vi "Main.vi"() -> ()   [LabVIEW 2017]
doc: "The program is for the real-time control of digital output pins on the Arduino Uno microcontroller.\n\nThe program is configured for the use of 6 DIO pins numbered 2-7. The pins can be be used to output AC and DC signals. The pins can also be swtiched on for a preset length of time."
uses:
  controls/UI Data.ctl
  <vilib>/MakerHub/LINX/Public/Peripherals/Digital/Digital Write 1 Chan.vi
  <vilib>/MakerHub/LINX/Public/Peripherals/Digital/Digital Write N Chans.vi
  <vilib>/MakerHub/LINX/Private/Local IO/LinxDigitalWrite.vi
  <vilib>/MakerHub/LINX/Public/Utilities/Check Channel.vi
  support/Message Queue/Enqueue Message (Single).vi
  <vilib>/MakerHub/LINX/Public/Utilities/Open Serial.vi
  <vilib>/MakerHub/LINX/Private/Utilties/Generate Error.vi
  <vilib>/Utility/error.llb/Error Cluster From Error Code.vi
  <vilib>/ErrorRing/Error Ring.xnode
  support/Message Queue/Message Queue.lvlib
  support/User Event - Stop/User Event - Stop.lvlib
  <vilib>/MakerHub/LINX/LMH-LINX.lvlib
panel:
  in  "Data Buffer":u64
  out "Playing Record":bool
  in  "Record New Sequence":bool
  in  "Play Button":bool
  in  "Previous Button":bool
  in  "Stop Button":bool
  in  "Next Button":bool
  in  "LG Electrodes":bool[][](array[boolean])=[[FALSE, FALSE], [FALSE, FALSE], [FALSE, FALSE]]
  in  "SM Electrodes":bool[][](array[boolean])=[[FALSE, FALSE, FALSE, FALSE, FALSE, FALSE], [FALSE, FALSE, FALSE, FALSE, FALSE, FALSE], [FALSE, FALSE, FALSE, FALSE, FALSE, FALSE], [FALSE, FALSE, FALSE, FALSE, FALSE, FALSE], [FALSE, FALSE, FALSE, FALSE, FALSE, FALSE], [FALSE, FALSE, FALSE, FALSE, FALSE, FALSE]]
  in  "XS Electrodes":bool[][](array[boolean])=[[FALSE, FALSE, FALSE], [FALSE, FALSE, FALSE], [FALSE, FALSE, FALSE], [FALSE, FALSE, FALSE], [FALSE, FALSE, FALSE], [FALSE, FALSE, FALSE]]
  in  "Frequency (Hz)":dbl
  in  "DC/AC":bool
  in  "On-time (ms)":dbl
  in  "Start Button":bool
  in  "COM Port":refnum<visa-resource-name>="COM3"
  out "User Prompts":string="Initializing...."
  in  "Restart Button":bool
  in  "Exit":bool
  # "Digital Microfluidics HV Switching Control"
  # "Electrode Recorded Sequence"
  # "Electrode Controls"
  # "Timing Controls"
  # "DC"
  # "AC"
  # "Program Status"
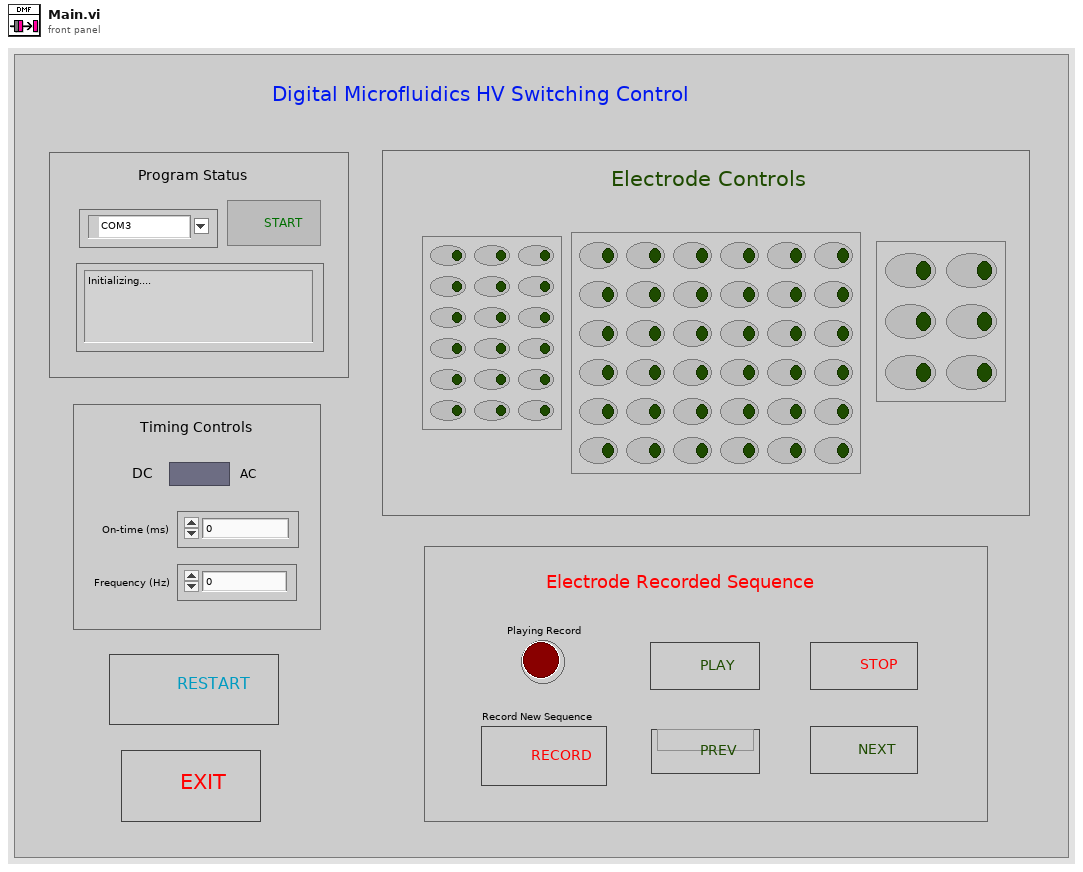
[diagram p1: front panel]
types:
  T1 = typedef "UI Data.ctl" = cluster{"VISA resource name":refnum<vi>, "Start Button":refnum<vi>, "DC/AC":refnum<vi>, "On-time (ms)":refnum<vi>, "Frequency (Hz)":refnum<vi>, "User Prompts":refnum<vi>, "XS Electrodes":refnum<vi>, "SM Electrodes":refnum<vi>, "LG Electrodes":refnum<vi>, "Data Buffer":refnum<vi>, "Play Button":refnum<vi>, "Playing Record":refnum<vi>, "Restart Button":refnum<vi>, "Exit":refnum<vi>}
  T2 = typedef "Message Queue.lvlib/All Message Queues.ctl" = cluster{"UI":refnum<queue>}
  T3 = typedef "LMH-LINX.lvlib/LINX Ref.ctl" = cluster{"IO":T4, "Interface":T5, "LINX Device Config":T6}
  T4 = typedef "LMH-LINX.lvlib/Platform.ctl" = enum16{"Remote", "Local"}
  T5 = typedef "LMH-LINX.lvlib/Interface.ctl" = enum16{"Serial", "TCP"}
  T6 = typedef "LMH-LINX.lvlib/Device.lvlib/LINX Device Config.ctl" = cluster{"Interface":T5, "COM Port":refnum<visa-resource-name>, "TCP Configuration":T7, "Device Family":u8, "Device ID":u8, "Device Name":string, "TCP Ref":refnum<k5>, "Channels":T8}
  T7 = typedef "LMH-LINX.lvlib/Device.lvlib/TCP Config.ctl" = cluster{"IP Address":string, "Port":u16}
  T8 = typedef "LMH-LINX.lvlib/Channels.ctl" = cluster{"DI":u8[], "DO":u8[], "AI":u8[], "AO":u8[], "PWM":u8[], "QE":u8[], "UART":u8[], "I2C 2":u8[], "SPI":u8[], "CAN":u8[], "Servo":u8[], "AI Ref (V)":dbl, "AI Resolution (Bits)":u8, "AO Ref (V)":dbl, "AO Resolution (Bits)":u8}
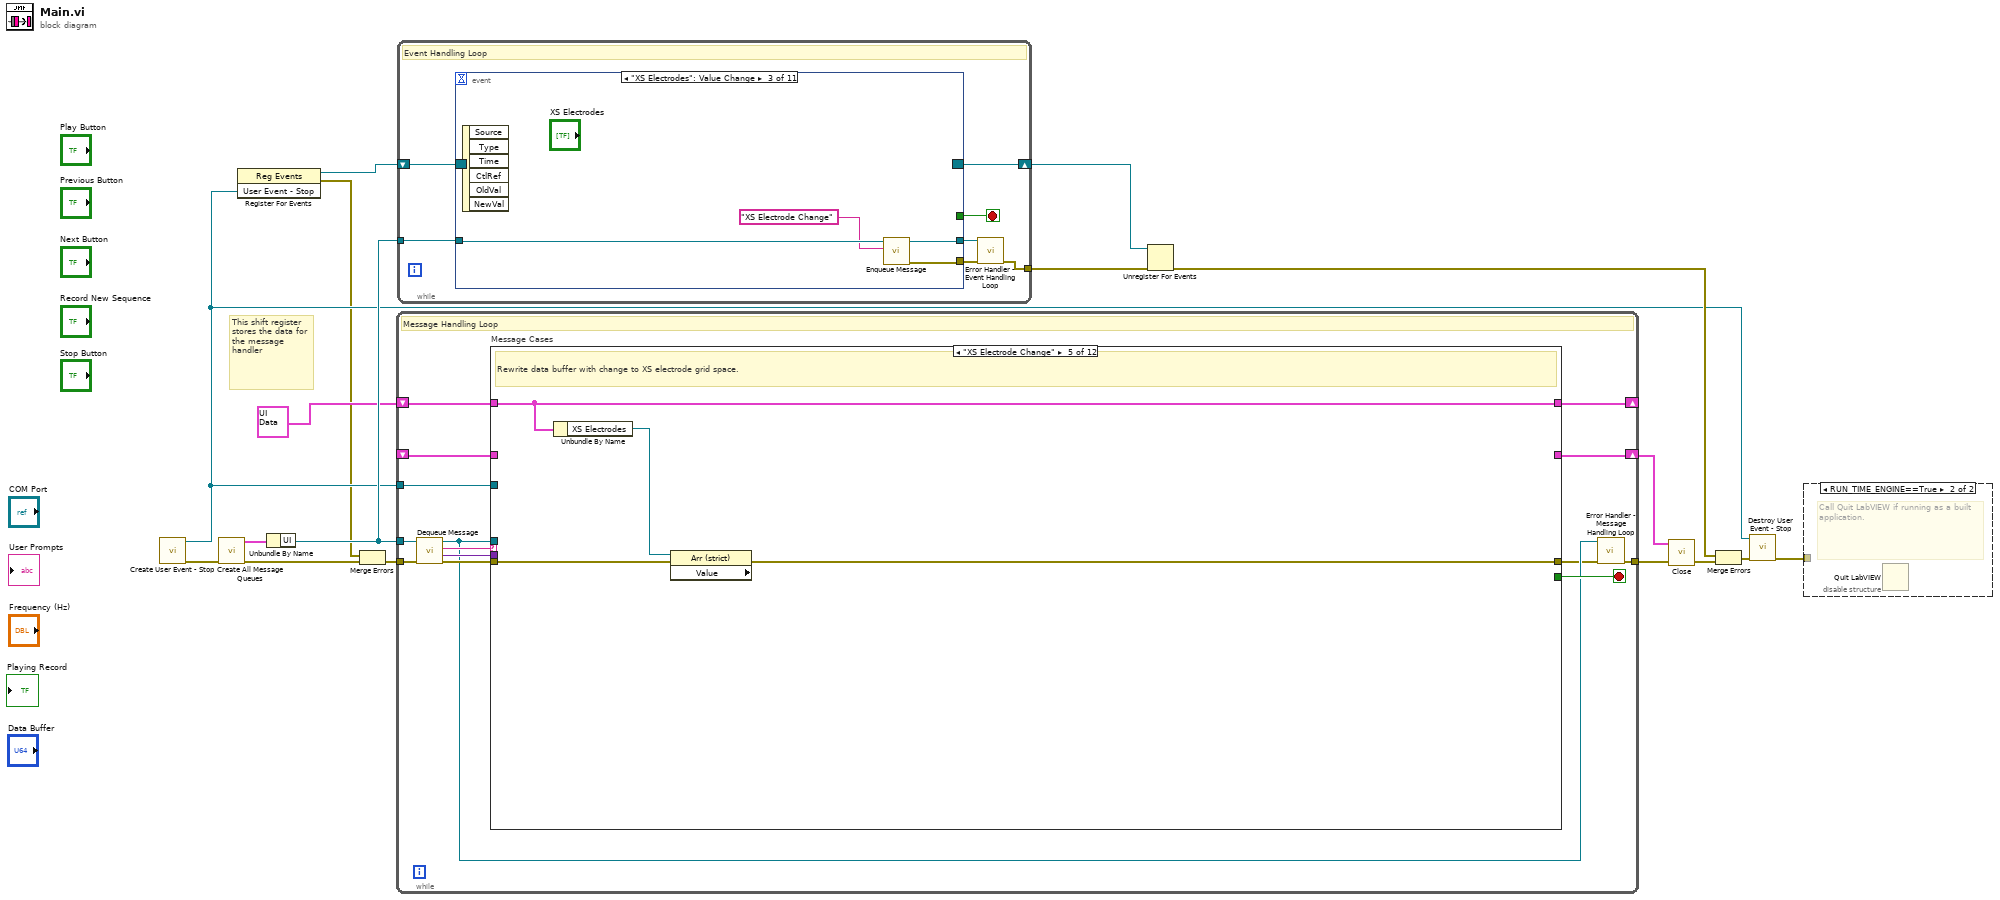
[diagram p0: block diagram]
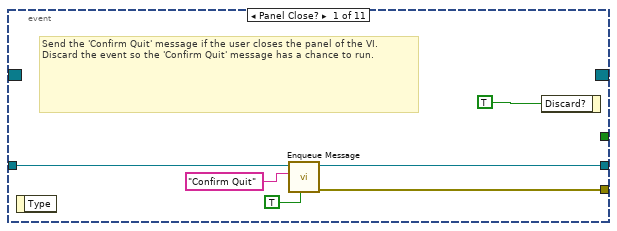
[diagram p3: hidden frame]
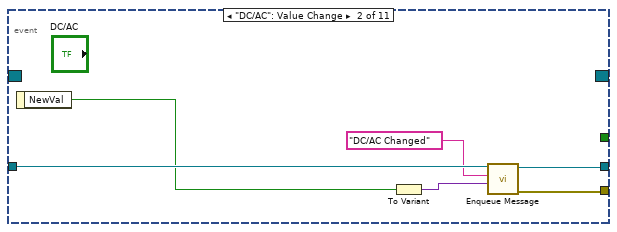
[diagram p4: hidden frame]
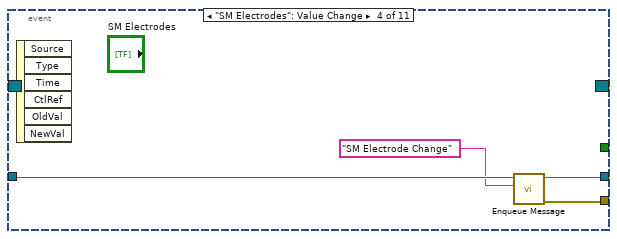
[diagram p5: hidden frame]
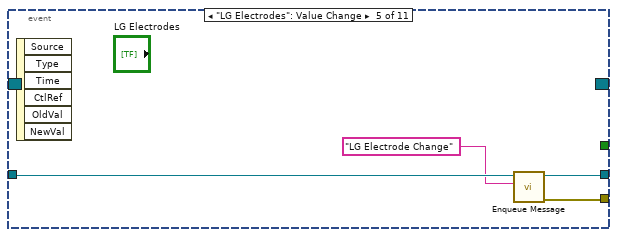
[diagram p6: hidden frame]
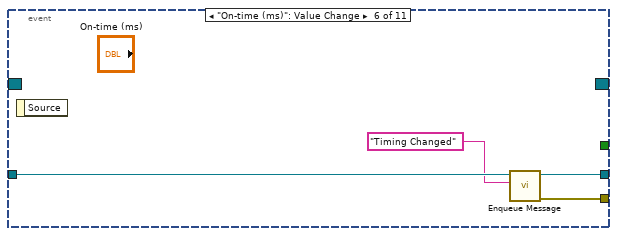
[diagram p7: hidden frame]
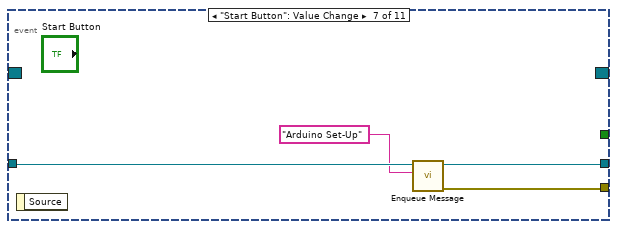
[diagram p8: hidden frame]
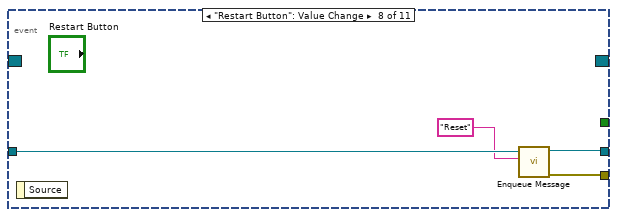
[diagram p9: hidden frame]
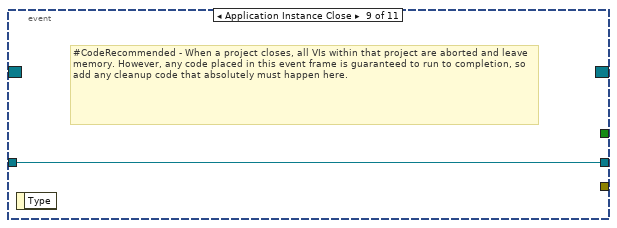
[diagram p10: hidden frame]
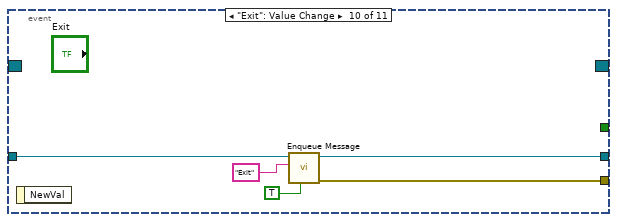
[diagram p11: hidden frame]
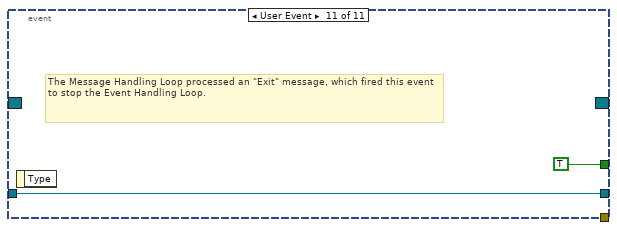
[diagram p12: hidden frame]
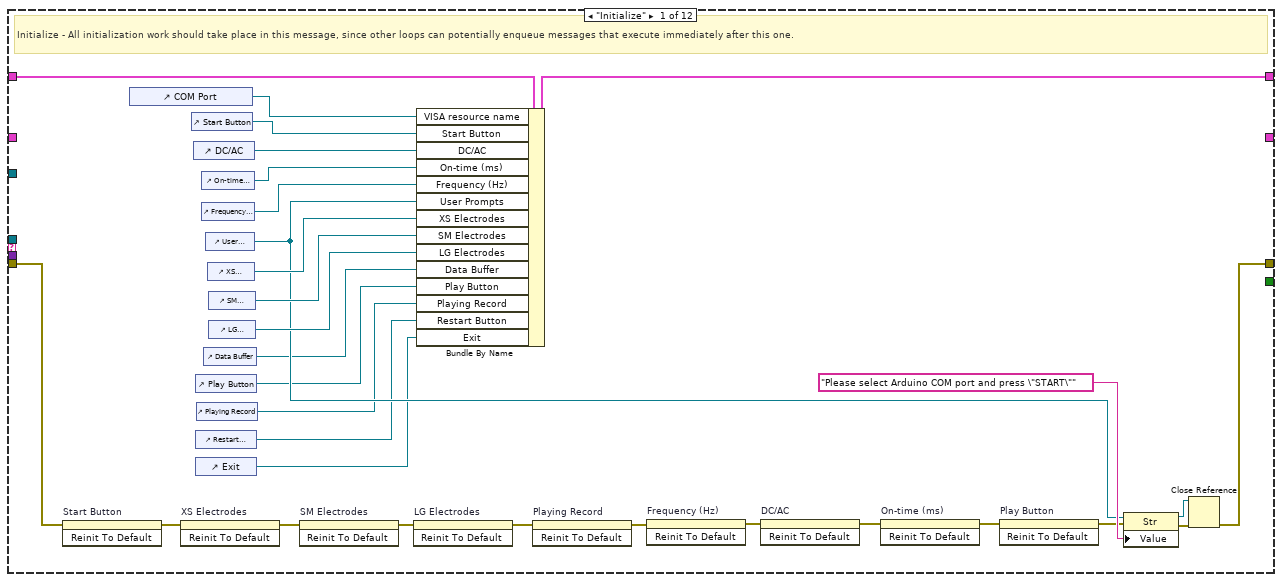
[diagram p13: hidden frame]
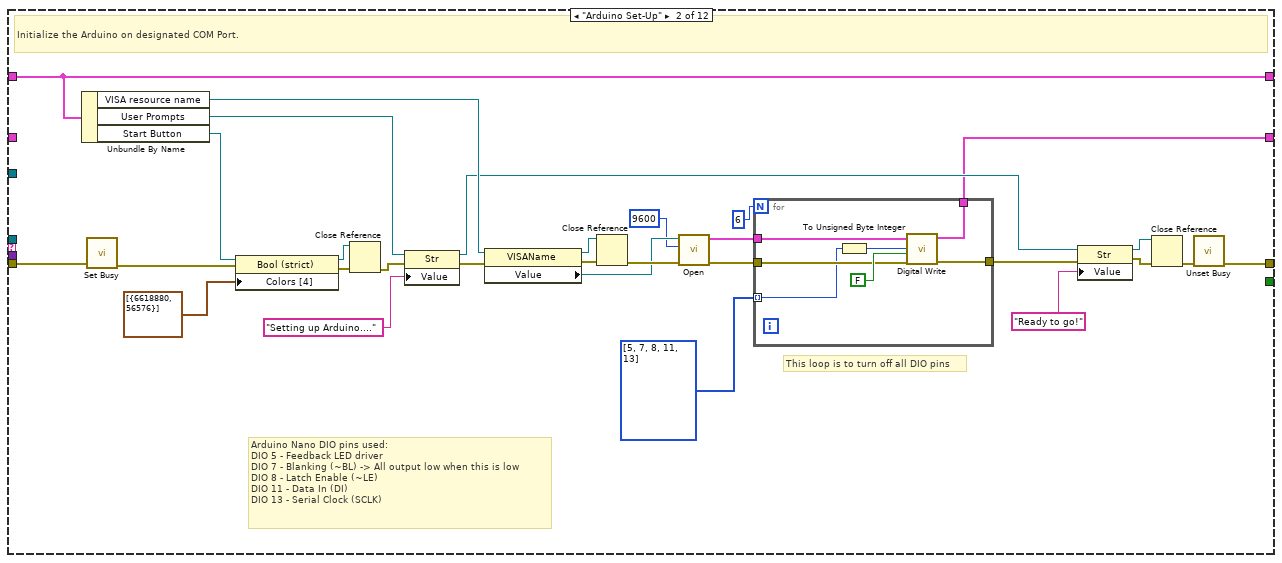
[diagram p14: hidden frame]
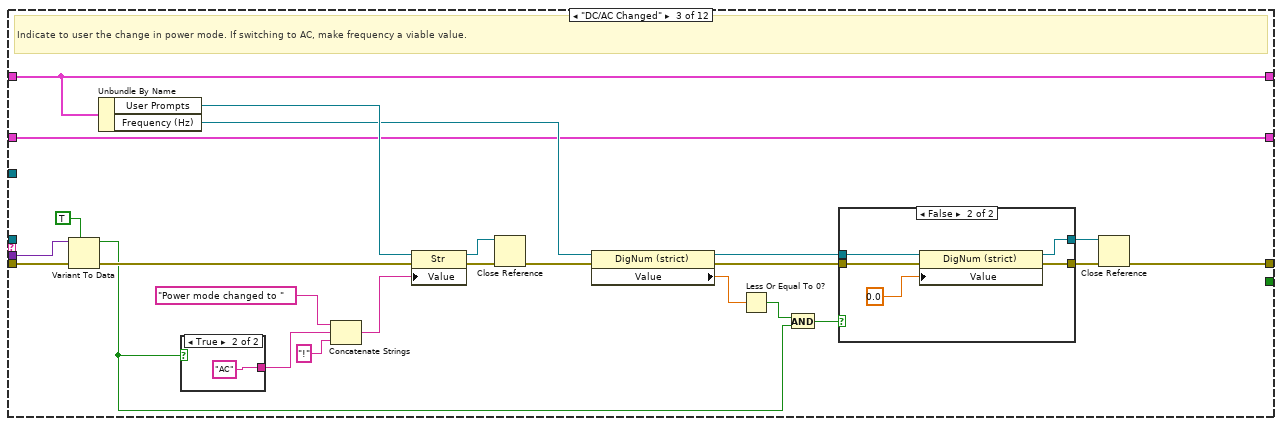
[diagram p15: hidden frame]
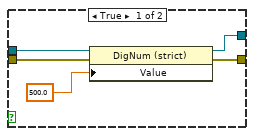
[diagram p16: hidden frame]
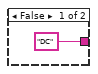
[diagram p17: hidden frame]
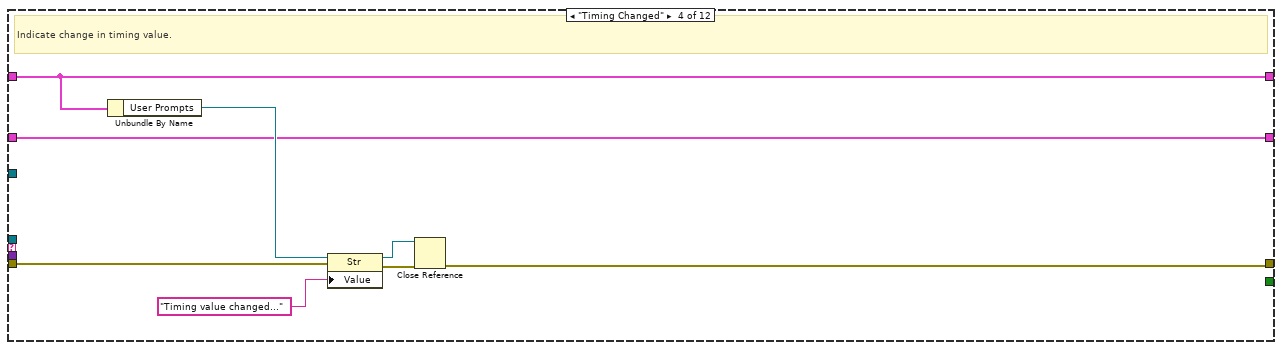
[diagram p18: hidden frame]
diagram:
  # "This shift register stores the data for the message handler"
  n1 = call "Create User Event - Stop.vi"() -> ("error out"=w14:errorcluster, "User Event - Stop"=w7:refnum<user-event>)  [unwired: 10 in]
  n2 = call "Create All Message Queues.vi"("error in (no error)"=w14) -> ("error out"=w17:errorcluster, "Message Queues out"=w16:T2)  [unwired: 9 in]
  n3 = register-events(w7) -> (reference out=w8:refnum<event-registration>, error out=w5:errorcluster)  [unwired: 2 in]
  n4 = Unbundle By Name(w16) -> ("UI"=w15:refnum<queue>)
  n5 = Merge Errors(w5, w17) -> (w6:errorcluster)
  n6 = while {
    tunnel: w15 -> [w23]
    shift-right: [w30] -> _
    shift-left: T1 {"VISA resource name"=refnum, "Start Button"=refnum, "DC/AC"=refnum, "On-time (ms)"=refnum, "Frequency (Hz)"=refnum, "User Prompts"=refnum, "XS Electrodes"=refnum, "SM Electrodes"=refnum, "LG Electrodes"=refnum, "Data Buffer"=refnum, "Play Button"=refnum, "Playing Record"=refnum, "Restart Button"=refnum, "Exit"=refnum} ("Data Cluster") -> [w31]
    tunnel: w7 -> [w28]
    tunnel: w6 -> [w27]
    tunnel: [w21] -> w3
    shift-right: [w19] -> w1
    shift-left: _ -> [w18]
    stop <- w29 stop-if-true
    # "Message Handling Loop"
    n7 = call "Dequeue Message.vi"("error in (no error)"=w27, "Message Queue"=w23) -> ("error out"=w26:errorcluster, "Message Data"=w24:variant, "Message"=w25:string, "dup Message Queue"=w22:refnum<queue>)  [unwired: 6 in]
    n8 = case "Message Cases" shown="\"XS Electrode Change\"" w25 {
      selector: w25 -> [_ _ _ _ _ _ _ _ _ _ _ w218]
      tunnel: w22 -> [_ _ _ _ _ _ _ w161 _ w191 w216 _]
      tunnel: w26 -> [w39 w81 w120 w140 w144 w147 w149 w154 w187 w195 w211 _]
      tunnel: [w55 w79 w100 w136 w142 w147 w149 w162 w181 w193 w214 w219] -> w20
      tunnel: w31 -> [w61 w90 w121 w141 w145 w146 w148 w170 w186 w194 w207 w220]
      tunnel: [w60 w90 w121 w141 w145 w146 w148 w170 w186 w194 w207 w220] -> w30
      tunnel: [_ _ _ _ _ _ _ _ _ _ TRUE _] -> w29
      tunnel: w24 -> [_ _ w119 _ _ _ _ _ w185 _ w208 _]
      tunnel: w28 -> [_ _ _ _ _ _ _ _ _ _ w213 _]
      tunnel: [_ w63 w98 w134 _ _ _ w150 w180 w188 w197 w217] -> w19
      tunnel: w18 -> [_ _ w98 w134 _ _ _ w168 w180 w188 w197 w217]
      frame "Initialize" {
        # "Initialize - All initialization work should take place in this message, since other loops can potentially enqueue messages that execute immediately after this one."
        n9 = invoke on="Start Button" class="Bool (strict)" method="Reinit To Default"(error in=w39) -> (error out=w47:errorcluster)  [unwired: 2 in, 2 out]
        n10 = control-ref of="COM Port"() -> (w59:refnum<vi>)
        n11 = invoke on="XS Electrodes" class="Arr (strict)" method="Reinit To Default"(error in=w47) -> (error out=w46:errorcluster)  [unwired: 2 in, 2 out]
        n12 = control-ref of="Start Button"() -> (w54:refnum<vi>)
        n13 = control-ref of="DC/AC"() -> (w52:refnum<vi>)
        n14 = control-ref of="Play Button"() -> (w35:refnum<vi>)
        n15 = control-ref of="Restart Button"() -> (w33:refnum<vi>)
        n16 = control-ref of="Exit"() -> (w32:refnum<vi>)
        n17 = control-ref of="Playing Record"() -> (w34:refnum<vi>)
        n18 = control-ref of="On-time (ms)"() -> (w51:refnum<vi>)
        n19 = control-ref of="Frequency (Hz)"() -> (w53:refnum<vi>)
        n20 = control-ref of="Data Buffer"() -> (w36:refnum<vi>)
        n21 = control-ref of="User Prompts"() -> (w37:refnum<vi>)
        n22 = control-ref of="XS Electrodes"() -> (w50:refnum<vi>)
        n23 = control-ref of="SM Electrodes"() -> (w49:refnum<vi>)
        n24 = control-ref of="LG Electrodes"() -> (w48:refnum<vi>)
        n25 = invoke on="SM Electrodes" class="Arr (strict)" method="Reinit To Default"(error in=w46) -> (error out=w45:errorcluster)  [unwired: 2 in, 2 out]
        n26 = invoke on="LG Electrodes" class="Arr (strict)" method="Reinit To Default"(error in=w45) -> (error out=w41:errorcluster)  [unwired: 2 in, 2 out]
        n27 = Bundle By Name(cluster=w61, "VISA resource name"=w59, "Start Button"=w54, "DC/AC"=w52, "On-time (ms)"=w51, "Frequency (Hz)"=w53, "User Prompts"=w37, "XS Electrodes"=w50, "SM Electrodes"=w49, "LG Electrodes"=w48, "Data Buffer"=w36, "Play Button"=w35, "Playing Record"=w34, "Restart Button"=w33, "Exit"=w32) -> (w60:T1)
        n28 = invoke on="Playing Record" class="Bool (strict)" method="Reinit To Default"(error in=w41) -> (error out=w40:errorcluster)  [unwired: 2 in, 2 out]
        n29 = invoke on="Frequency (Hz)" class="DigNum (strict)" method="Reinit To Default"(error in=w40) -> (error out=w44:errorcluster)  [unwired: 2 in, 2 out]
        n30 = invoke on="DC/AC" class="Bool (strict)" method="Reinit To Default"(error in=w44) -> (error out=w43:errorcluster)  [unwired: 2 in, 2 out]
        n31 = invoke on="On-time (ms)" class="DigNum (strict)" method="Reinit To Default"(error in=w43) -> (error out=w42:errorcluster)  [unwired: 2 in, 2 out]
        n32 = invoke on="Play Button" class="Bool" method="Reinit To Default"(error in=w42) -> (error out=w38:errorcluster)  [unwired: 2 in, 2 out]
        n33 = property class="Str"(reference=w37, error in=w38, "Value"="Please select Arduino COM port and press \"START\"") -> (reference out=w57:refnum<vi>, error out=w58:errorcluster)
        n34 = Close Reference(reference=w57, error in (no error)=w58) -> (error out=w55:errorcluster)
      }
      frame "Arduino Set-Up" {
        # "Arduino Nano DIO pins used:\nDIO 5 - Feedback LED driver\nDIO 7 - Blanking (~BL) -> All output low when this is low\nDIO 8 - Latch Enable (~LE)\nDIO 11 - Data In (DI)\nDIO 13 - Serial Clock (SCLK)"
        # "This loop is to turn off all DIO pins"
        # "Initialize the Arduino on designated COM Port."
        n35 = Unbundle By Name(w90) -> ("VISA resource name"=w89:refnum<vi>, "User Prompts"=w83:refnum<vi>, "Start Button"=w72:refnum<vi>)
        n36 = call <vilib>:"Set Busy.vi"("error in (no error)"=w81) -> ("error out"=w73:errorcluster)  [unwired: 9 in, 1 out]
        n37 = property class="Bool (strict)"(reference=w72, error in=w73, "Colors [4]"=cluster{u32, u32}[] [{6618880, 56576}]) -> (reference out=w68:refnum<vi>, error out=w70:errorcluster)
        n38 = Close Reference(reference=w68, error in (no error)=w70) -> (error out=w69:errorcluster)
        n39 = property class="Str"(reference=w83, error in=w69, "Value"="Setting up Arduino....") -> (reference out=w77:refnum<vi>, error out=w78:errorcluster)
        n40 = property class="VISAName"(reference=w89, error in=w78) -> (reference out=w87:refnum<vi>, error out=w88:errorcluster, "Value"=w75:refnum<visa-resource-name>)
        n41 = Close Reference(reference=w87, error in (no error)=w88) -> (error out=w76:errorcluster)
        n42 = call-poly <vilib>:"Open.vi"("Error In"=w76, "Baud Rate Override"=u32 9600, "Serial Port"=w75) -> ("Error Out"=w66:errorcluster, "LINX Resource"=w64:T3)  [unwired: 6 in, 1 out]
        n43 = for {
          N: 6 -> [_]
          tunnel: [w97] -> w65
          tunnel: [w95] -> w63
          tunnel: w66 -> [w94]
          tunnel: w64 -> [w93]
          tunnel: u8[] [5, 7, 8, 11, 13] -> [w91] mode=indexing
          n44 = To Unsigned Byte Integer(number=w91) -> (unsigned 8bit integer=w92:u8)
          n45 = call-poly <vilib>:"Digital Write.vi"("Error In"=w94, "Output Value"=FALSE, "DO Channel"=w92, "LINX Resource"=w93) -> ("Error Out"=w97:errorcluster, "LINX Resource"=w95:T3)  [unwired: 6 in]
        }
        n46 = property class="Str"(reference=w77, error in=w65, "Value"="Ready to go!") -> (reference out=w85:refnum<vi>, error out=w86:errorcluster)
        n47 = Close Reference(reference=w85, error in (no error)=w86) -> (error out=w80:errorcluster)
        n48 = call <vilib>:"Unset Busy.vi"("error in (no error)"=w80) -> ("error out"=w79:errorcluster)  [unwired: 10 in]
      }
      frame "DC/AC Changed" {
        # "Indicate to user the change in power mode. If switching to AC, make frequency a viable value."
        n49 = Variant To Data(error in=w120, type=TRUE, Variant=w119) -> (data=w105:bool, error out=w115:errorcluster)
        n50 = Unbundle By Name(w121) -> ("User Prompts"=w112:refnum<vi>, "Frequency (Hz)"=w108:refnum<vi>)
        n51 = case shown="True" w105 {
          tunnel: ["DC" "AC"] -> w116
          frame False {
          }
          frame True {
          }
        }
        n52 = Concatenate Strings("Power mode changed to " ("string"), w116, "!") -> (w111:string)
        n53 = property class="Str"(reference=w112, error in=w115, "Value"=w111) -> (reference out=w113:refnum<vi>, error out=w114:errorcluster)
        n54 = Close Reference(reference=w113, error in (no error)=w114) -> (error out=w109:errorcluster)
        n55 = property class="DigNum (strict)"(reference=w108, error in=w109) -> (reference out=w102:refnum<vi>, error out=w103:errorcluster, "Value"=w107:dbl)
        n56 = Less Or Equal To 0?(x=w107) -> (x <= 0?=w106:bool)
        n57 = And(x=w106, y=w105) -> (x .and. y?=w104:bool)
        n58 = case shown="False" w104 {
          tunnel: w103 -> [w126 w131]
          tunnel: w102 -> [w125 w130]
          tunnel: [w123 w128] -> w101
          tunnel: [w122 w127] -> w99
          frame True {
            n59 = property class="DigNum (strict)"(reference=w125, error in=w126, "Value"=500.0) -> (reference out=w122:refnum<vi>, error out=w123:errorcluster)
          }
          frame False {
            n60 = property class="DigNum (strict)"(reference=w130, error in=w131, "Value"=0.0) -> (reference out=w127:refnum<vi>, error out=w128:errorcluster)
          }
        }
        n61 = Close Reference(reference=w99, error in (no error)=w101) -> (error out=w100:errorcluster)
      }
      frame "Timing Changed" {
        # "Indicate change in timing value."
        n62 = Unbundle By Name(w141) -> ("User Prompts"=w139:refnum<vi>)
        n63 = property class="Str"(reference=w139, error in=w140, "Value"="Timing value changed...") -> (reference out=w137:refnum<vi>, error out=w138:errorcluster)
        n64 = Close Reference(reference=w137, error in (no error)=w138) -> (error out=w136:errorcluster)
      }
      frame "XS Electrode Change" {
        # "Rewrite data buffer with change to XS electrode grid space."
        n65 = Unbundle By Name(w145) -> ("XS Electrodes"=w143:refnum<vi>)
        n66 = property class="Arr (strict)" props=["Value"](reference=w143, error in=w144) -> (error out=w142:errorcluster)  [unwired: 2 out]
      }
      frame "SM Electrode Change" {
        # "Rewrite data buffer with change to SM electrode grid space."
      }
      frame "LG Electrode Change" {
        # "Rewrite data buffer with change to LG electrode grid space."
      }
      frame "Reset" {
        # "Set start button colour back to intial grey"
        # "This loop is to turn off all DIO pins"
        # "Turn all DIO pins off, reset front element features which are not covered by initialization. After clean-up, return to initialization."
        n67 = Unbundle By Name(w170) -> ("Start Button"=w164:refnum<vi>, "User Prompts"=w157:refnum<vi>)
        n68 = call <vilib>:"Set Busy.vi"("error in (no error)"=w154) -> ("error out"=w153:errorcluster)  [unwired: 9 in, 1 out]
        n69 = property class="Str"(reference=w157, error in=w153, "Value"="Reseting... Please Wait...") -> (reference out=w156:refnum<vi>, error out=w159:errorcluster)
        n70 = Close Reference(reference=w156, error in (no error)=w159) -> (error out=w158:errorcluster)
        n71 = for {
          N: 6 -> [_]
          tunnel: [w179] -> w165
          tunnel: [w177] -> w150
          tunnel: w158 -> [w174]
          tunnel: w168 -> [w173]
          i -> [w176]
          n72 = Add(x=2, y=w176) -> (x+y=w171:i32)
          n73 = To Unsigned Byte Integer(number=w171) -> (unsigned 8bit integer=w172:u8)
          n74 = call-poly <vilib>:"Digital Write.vi"("Error In"=w174, "Output Value"=FALSE, "DO Channel"=w172, "LINX Resource"=w173) -> ("Error Out"=w179:errorcluster, "LINX Resource"=w177:T3)  [unwired: 6 in]
        }
        n75 = property class="Bool (strict)"(reference=w164, error in=w165, "Colors [4]"=cluster{u32, u32}[] [{12369084, 12369084}, {6618880, 56576}]) -> (reference out=w163:refnum<vi>, error out=w167:errorcluster)
        n76 = Close Reference(reference=w163, error in (no error)=w167) -> (error out=w151:errorcluster)
        n77 = call <vilib>:"Unset Busy.vi"("error in (no error)"=w151) -> ("error out"=w152:errorcluster)  [unwired: 10 in]
        n78 = call-poly "Enqueue Message.vi"("error in (no error)"=w152, "Message"="Initialize", "Message Queue"=w161) -> ("error out"=w162:errorcluster)  [unwired: 7 in, 1 out]
      }
      frame "Error" {
        # "#CodeRecommended - If you ever change the name of this \"Error\" message, you'll need to update the name in the Check Loop Error.vi as well."
        # "#CodeRecommended - Consider creating a system for logging errors in some way. These errors are for notification purposes only. Handling of specific errors should be performed in the message frames that generated the error."
        # "Error - Display an error dialog. This message is sent by the \"Error Handler\" VIs at the end of other loops in this application."
        n79 = Variant To Data(error in=w187, type=errorcluster {"status"=FALSE, "code"=0, "source"=""} ("error constant"), Variant=w185) -> (data=w183:errorcluster, error out=w182:errorcluster)
        n80 = call <vilib>:"Simple Error Handler.vi"("error in (no error)"=w183) -> ()  [unwired: 4 in, 5 out]
        n81 = Merge Errors(w182) -> (w181:errorcluster)
      }
      frame "Confirm Quit" {
        # "#CodeNeeded - If you want to provide an \"Are you sure\" dialog (or some other notification) before the application exits, place that code here. This message is typically sent from a Panel Close? event."
        # "Confirm Quit - Message that can confirm whether or not the user wants to exit the application."
        n82 = call-poly "Enqueue Message.vi"("Priority Message? (F)"=TRUE, "error in (no error)"=w195, "Message"="Exit", "Message Queue"=w191) -> ("error out"=w192:errorcluster)  [unwired: 6 in, 1 out]
        n83 = Merge Errors(w192) -> (w193:errorcluster)
      }
      frame "Exit" {
        # "Stop the VI"
        # "Release the message queue reference"
        # "Exit - Exit the application. Clean up by setting the start button back to original colours. Also turn off all digital output pins on arduino."
        n84 = Variant To Data(type=errorcluster {"status"=FALSE, "code"=0, "source"=""} ("error constant"), Variant=w208) -> (data=w209:errorcluster)  [unwired: 1 in, 1 out]
        n85 = call <vilib>:"Simple Error Handler.vi"("error in (no error)"=w209) -> ()  [unwired: 4 in, 5 out]
        n86 = Unbundle By Name(w207) -> ("XS Electrodes"=w199:refnum<vi>, "Start Button"=w202:refnum<vi>)
        n87 = call "Fire User Event - Stop.vi"("User Event - Stop"=w213) -> ("error out"=w212:errorcluster)  [unwired: 10 in]
        n88 = Release Queue(queue=w216, error in (no error)=w211) -> (error out=w206:errorcluster)  [unwired: 1 in, 2 out]
        n89 = property class="Bool (strict)"(reference=w202, error in=w206, "Colors [4]"=cluster{u32, u32}[] [{12369084, 12369084}, {6618880, 56576}]) -> (reference out=w204:refnum<vi>, error out=w205:errorcluster)
        n90 = Close Reference(reference=w204, error in (no error)=w205) -> (error out=w196:errorcluster)
        n91 = invoke class="Arr (strict)" method="Reinit To Default"(reference=w199, error in=w196) -> (reference out=w198:refnum<vi>, error out=w201:errorcluster)  [unwired: 1 in, 1 out]
        n92 = Close Reference(reference=w198, error in (no error)=w201) -> (error out=w200:errorcluster)
        n93 = Merge Errors(w212, w200) -> (w214:errorcluster)
      }
      frame Default {
        # "'Default' case only runs if there is a message that isn't defined in any of the other cases.  Output a programming error."
        n94 = xnode "Error Ring"("parameter 0"=w218) -> ("error out"=w219:errorcluster)
      }
    }
    n95 = call "Error Handler - Message Handling Loop.vi"("error in (no error)"=w20, "Message Queue"=w22) -> ("dup error in"=w21:errorcluster)  [unwired: 8 in, 1 out]
  }
  n96 = while {
    tunnel: w15 -> [w234]
    shift-right: [w232] -> w11
    shift-left: w8 -> [w233]
    tunnel: [w228] -> w9
    stop <- w230 stop-if-true
    # "Event Handling Loop"
    n97 = event shown="[2] \"XS Electrodes\": Value Change" {
      selector: w233 -> [_ _ _ _ _ _ _ _ _ _ _]
      dyn-events: [_ _ _ _ _ _ _ _ _ _ _] -> w232
      timeout: _ -> [_ _ _ _ _ _ _ _ _ _ _]
      tunnel: [_ _ _ _ _ _ _ _ _ _ TRUE ("Discard?")] -> w230
      tunnel: w234 -> [w239 w245 w248 w252 w256 w260 w265 w270 w271 w276 w278]
      tunnel: [w238 w246 w249 w253 w257 w261 w264 w268 _ w275 _] -> w231
      tunnel: [w237 w244 w250 w254 w258 w262 w266 w269 w271 w274 w278] -> w229
      event Panel Close? {
        # "Send the 'Confirm Quit' message if the user closes the panel of the VI. Discard the event so the 'Confirm Quit' message has a chance to run."
        n98 = event-data() -> ()  [unwired: 1 in, 1 out]
        n99 = call-poly "Enqueue Message.vi"("Priority Message? (F)"=TRUE, "Message"="Confirm Quit", "Message Queue"=w239) -> ("error out"=w238:errorcluster, "dup Message Queue"=w237:refnum<queue>)  [unwired: 7 in]
        n100 = event-data("Discard?"=TRUE) -> ()  [unwired: 1 in, 1 out]
      }
      event "DC/AC": Value Change {
        n101 = event-data() -> ("NewVal"=w243:bool)  [unwired: 1 in]
        n102 = To Variant(anything=w243) -> (Variant=w242:variant)
        n103 = call-poly "Enqueue Message.vi"("Message Data"=w242, "Message"="DC/AC Changed", "Message Queue"=w245) -> ("error out"=w246:errorcluster, "dup Message Queue"=w244:refnum<queue>)  [unwired: 7 in]
      }
      event "XS Electrodes": Value Change {
        n104 = event-data() -> ()  [unwired: 1 in, 6 out]
        n105 = call-poly "Enqueue Message.vi"("Message"="XS Electrode Change", "Message Queue"=w248) -> ("error out"=w249:errorcluster, "dup Message Queue"=w250:refnum<queue>)  [unwired: 8 in]
      }
      event "SM Electrodes": Value Change {
        n106 = event-data() -> ()  [unwired: 1 in, 6 out]
        n107 = call-poly "Enqueue Message.vi"("Message"="SM Electrode Change", "Message Queue"=w252) -> ("error out"=w253:errorcluster, "dup Message Queue"=w254:refnum<queue>)  [unwired: 8 in]
      }
      event "LG Electrodes": Value Change {
        n108 = event-data() -> ()  [unwired: 1 in, 6 out]
        n109 = call-poly "Enqueue Message.vi"("Message"="LG Electrode Change", "Message Queue"=w256) -> ("error out"=w257:errorcluster, "dup Message Queue"=w258:refnum<queue>)  [unwired: 8 in]
      }
      event "On-time (ms)": Value Change {
        n110 = event-data() -> ()  [unwired: 1 in, 1 out]
        n111 = call-poly "Enqueue Message.vi"("Message"="Timing Changed", "Message Queue"=w260) -> ("error out"=w261:errorcluster, "dup Message Queue"=w262:refnum<queue>)  [unwired: 8 in]
      }
      event "Start Button": Value Change {
        n112 = event-data() -> ()  [unwired: 1 in, 1 out]
        n113 = call-poly "Enqueue Message.vi"("Message"="Arduino Set-Up", "Message Queue"=w265) -> ("error out"=w264:errorcluster, "dup Message Queue"=w266:refnum<queue>)  [unwired: 8 in]
      }
      event "Restart Button": Value Change {
        n114 = event-data() -> ()  [unwired: 1 in, 1 out]
        n115 = call-poly "Enqueue Message.vi"("Message"="Reset", "Message Queue"=w270) -> ("error out"=w268:errorcluster, "dup Message Queue"=w269:refnum<queue>)  [unwired: 8 in]
      }
      event Application Instance Close {
        # "#CodeRecommended - When a project closes, all VIs within that project are aborted and leave memory. However, any code placed in this event frame is guaranteed to run to completion, so add any cleanup code that absolutely must happen here."
        n116 = event-data() -> ()  [unwired: 1 in, 1 out]
      }
      event "Exit": Value Change {
        n117 = event-data() -> ()  [unwired: 1 in, 1 out]
        n118 = call-poly "Enqueue Message.vi"("Priority Message? (F)"=TRUE, "Message"="Exit", "Message Queue"=w276) -> ("error out"=w275:errorcluster, "dup Message Queue"=w274:refnum<queue>)  [unwired: 7 in]
      }
      event User Event {
        # "The Message Handling Loop processed an \"Exit\" message, which fired this event to stop the Event Handling Loop."
        n119 = event-data() -> ()  [unwired: 1 in, 1 out]
      }
    }
    n120 = call "Error Handler - Event Handling Loop.vi"("error in (no error)"=w231, "Message Queue"=w229) -> ("dup error in"=w228:errorcluster)  [unwired: 8 in, 1 out]
  }
  n121 = Unregister For Events(event registration refnum=w11, error in=w9) -> (error out=w12:errorcluster)
  n122 = call <vilib>:"Close.vi"("Error In"=w3, "LINX Resource"=w1) -> ("Error Out"=w2:errorcluster)  [unwired: 9 in]
  n123 = Merge Errors(w12, w2) -> (w13:errorcluster)
  n124 = call "Destroy User Event - Stop.vi"("error in (no error)"=w13, "User Event - Stop"=w7) -> ("error out"=w4:errorcluster)  [unwired: 9 in]
  n125 = disable-structure shown="RUN_TIME_ENGINE==True" {
    disable-tunnel: w4 -> [_ _]
    frame condition #0 (active) {
    }
    frame condition #1 {
      # "Call Quit LabVIEW if running as a built application."
      n126 = Quit LabVIEW() -> ()  [unwired: 1 in]
    }
  }
